vi "Read Schema.vi"(8 "error in (no error)":errorcluster, 11 "FE FF Frame in":refnum<class "FE FF Frame.lvclass">) -> (0 "error out":errorcluster, 2 "Schema":string, 3 "FE FF Frame out":refnum<class "FE FF Frame.lvclass">)   [LabVIEW 2023, in "Data Analysis.lvlib" / "FE FF Frame.lvlib" / "FE FF Frame.lvclass"]
uses:
  FE FF Frame.lvclass
  FE FF Frame.lvclass/FE FF Frame.ctl
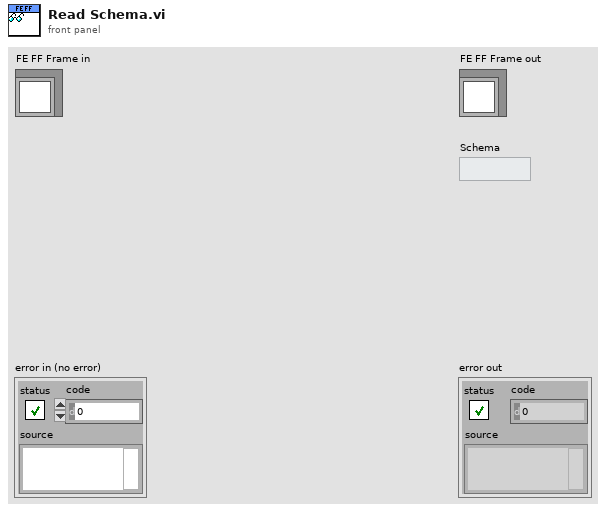
[diagram p1: front panel]
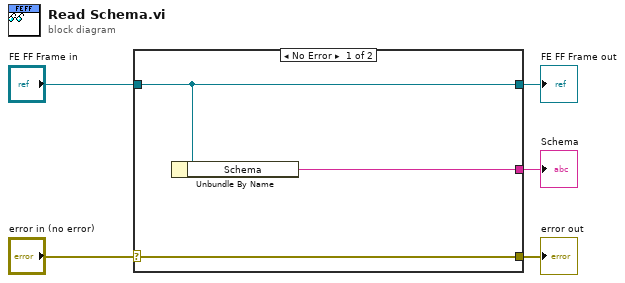
[diagram p0: block diagram]
diagram:
  n1 = case shown="No Error" "error in (no error)" {
    selector: "error in (no error)" -> [w8 w9]
    tunnel: [w8 w9] -> w4
    tunnel: [w7 w10] -> w2
    tunnel: "FE FF Frame in" -> [w7 w10]
    tunnel: [w6 _] -> w1
    frame No Error {
      n2 = Unbundle By Name(w7) -> ("Schema"=w6:string)
    }
    frame Error {
    }
  }
  "error out" <- w4
  "FE FF Frame out" <- w2
  "Schema" <- w1
